vi "JSON to LVObject - Aggregate - Returns Matching Types.vi"() -> ()   [LabVIEW 2017, in "Tests.lvlib" / "Type Name Handling.lvlib"]
uses:
  Flatten To JSON Object/Flatten To JSON Object.lvclass
  City/City.lvclass
  Flatten To JSON Object/Type Name Handling.ctl
  Flatten To JSON Object/Flatten To JSON Object.lvclass/Flatten To JSON Object.ctl
  Flatten To JSON Object/Write Type Name Handling.vi
  Temperature Forecast/Temperature Forecast.lvclass
  C:/Users/de200256/Code/logmanoriginal/jsontext-object-serialization/Tests/Weather Forecast/Weather Forecast.lvclass
  <vilib>/addons/_JKI Toolkits/Caraya/classes/Assert/Assert Equal Value and Type_Variant.vi
  Type Name Handling.lvlib
  <vilib>/addons/_JKI Toolkits/Caraya/classes/Test/Test.lvclass
  <vilib>/addons/_JKI Toolkits/Caraya/classes/Assert/Assert.lvclass
panel:
  out "error out":errorcluster
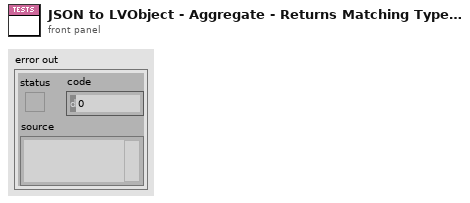
[diagram p1: front panel]
types:
  T1 = typedef "Flatten To JSON Object.lvclass/Type Name Handling.ctl" = enum16{"None", "Inline"}
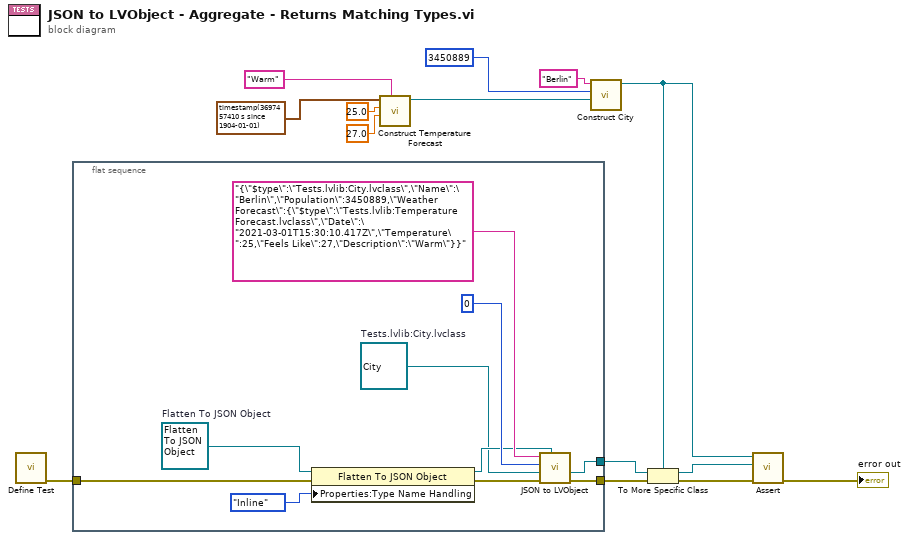
[diagram p0: block diagram]
diagram:
  n1 = call <vilib>:"Define Test.vi"() -> ("error out"=w14:errorcluster)  [unwired: 11 in]
  n2 = flat-sequence {
    tunnel: w14 -> [w24]
    tunnel: [w16] -> w5
    tunnel: [w15] -> w4
    frame #0 {
      w17 = refnum<class "City.lvclass"> refnum  # Tests.lvlib:City.lvclass
      w20 = refnum<class "Flatten To JSON Object.lvclass"> refnum  # Flatten To JSON Object
      n3 = property class="Flatten To JSON Object"(reference=w20, error in=w24, "Properties:Type Name Handling"=Type_Name_Handling."Inline" ("Type Name Handling")) -> (reference out=w19:refnum<class "Flatten To JSON Object.lvclass">, error out=w21:errorcluster)
      n4 = call-dynamic "JSON to LVObject.vi"("Flatten To JSON Object in"=w19, "error in (no error)"=w21, "Object Type"=w17, "Offset"=0, "JSON"="{\"$type\":\"Tests.lvlib:City.lvclass\",\"Name\":\"Berlin\",\"Population\":3450889,\"Weather Forecast\":{\"$type\":\"Tests.lvlib:Temperature Forecast.lvclass\",\"Date\":\"2021-03-01T15:30:10.417Z\",\"Temperature\":25,\"Feels Like\":27,\"Description\":\"Warm\"}}") -> ("error out"=w15:errorcluster, "Object"=w16:refnum<class>)  [unwired: 5 in]
    }
  }
  n5 = call "Construct Temperature Forecast.vi"("Description"="Warm", "Feels Like [°C]"=27.0, "Temperature [°C]"=25.0, "Date"=timestamp(3697457410.417 s since 1904-01-01)) -> ("Temperature Forecast"=w6:refnum<class "Temperature Forecast.lvclass">)  [unwired: 6 in, 1 out]
  n6 = call "Construct City.vi"("Weather Forecast"=w6, "Population"=u32 3450889, "Name"="Berlin") -> ("City"=w1:refnum<class "City.lvclass">)  [unwired: 7 in, 1 out]
  n7 = To More Specific Class(target class=w1, reference=w5, error in=w4) -> (specific class reference=w3:refnum<class "City.lvclass">, error out=w2:errorcluster)
  n8 = call-poly <vilib>:"Assert.vi"("error in (no error)"=w2, "Y"=w3, "X"=w1) -> ("error out"=→"error out":errorcluster)  [unwired: 8 in]
